vi "JKI_Python_Server Example 2 Nodes.vi"() -> ()   [LabVIEW 2013]
uses:
  Server/Type Definitions/Python Method.ctl
  Server/Register for Events (Single PyObject).vi
  Server/Server.lvclass
  Call/Call.lvclass
panel:
  out "Number of Connections":u32
  out "Client Connected":bool
  out "error out":errorcluster
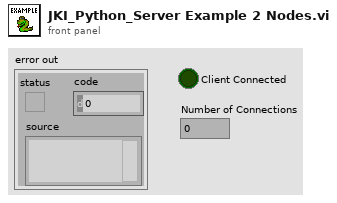
[diagram p1: front panel]
types:
  T1 = typedef "JKI_Python_Bridge_for_LV.lvlib/Server.lvclass/Python Method.ctl" = cluster{"Name":string, "Arguments":string[], "Documentation":string}
  T2 = typedef "JKI_Python_Bridge_for_LV.lvlib/Server.lvclass/Python Method Call - Event Registration.ctl" = refnum<event-registration>
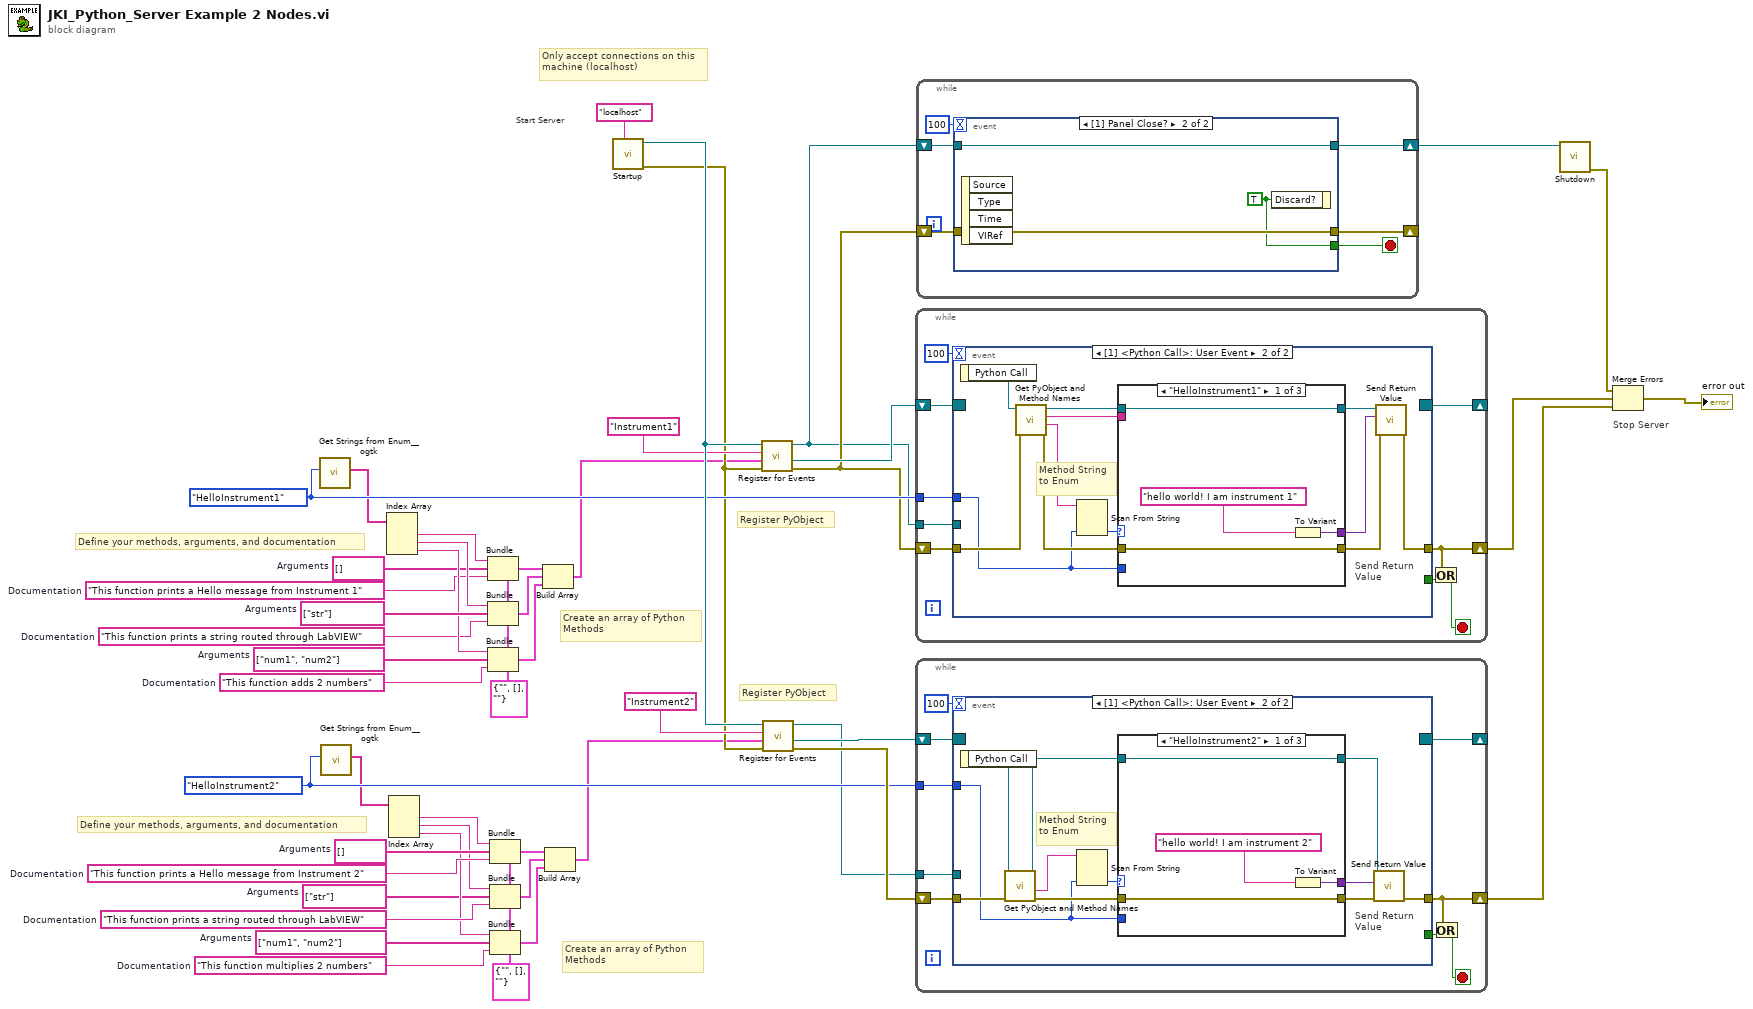
[diagram p0: block diagram]
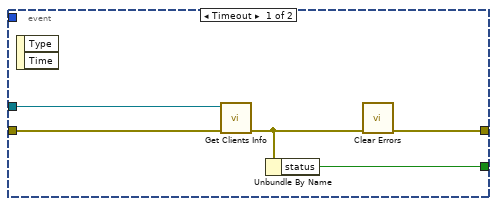
[diagram p2: hidden frame]
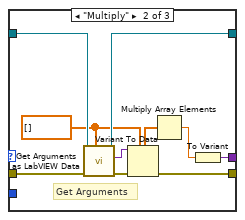
[diagram p3: hidden frame]
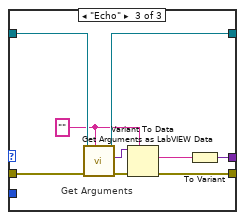
[diagram p4: hidden frame]
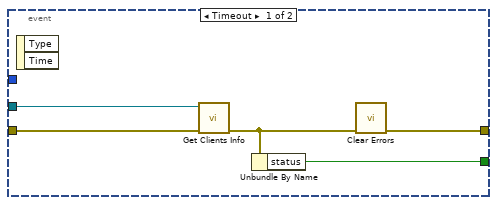
[diagram p5: hidden frame]
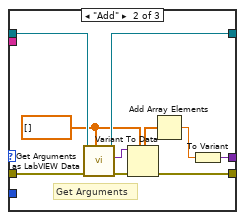
[diagram p6: hidden frame]
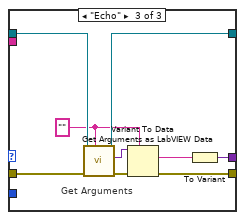
[diagram p7: hidden frame]
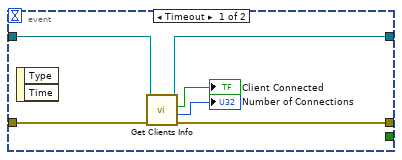
[diagram p8: hidden frame]
diagram:
  w15 = string[] []  # Arguments
  w14 = T1 {"Name"="", "Arguments"=[], "Documentation"=""} ("Method")
  w13 = "This function multiplies 2 numbers"  # Documentation
  w12 = "This function prints a string routed through LabVIEW"  # Documentation
  w11 = "This function prints a Hello message from Instrument 2"  # Documentation
  w6 = string[] ["num1", "num2"]  # Arguments
  w5 = string[] ["str"]  # Arguments
  w18 = string[] []  # Arguments
  w19 = T1 {"Name"="", "Arguments"=[], "Documentation"=""} ("Method")
  w20 = "This function adds 2 numbers"  # Documentation
  w21 = "This function prints a string routed through LabVIEW"  # Documentation
  w22 = "This function prints a Hello message from Instrument 1"  # Documentation
  w27 = string[] ["num1", "num2"]  # Arguments
  w28 = string[] ["str"]  # Arguments
  w40 = enum16{"HelloInstrument2", "Echo", "Multiply"}."HelloInstrument2"
  w39 = enum16{"HelloInstrument1", "Echo", "Add"}."HelloInstrument1"
  # "Create an array of Python \nMethods"
  # "Define your methods, arguments, and documentation"
  # "Create an array of Python \nMethods"
  # "Define your methods, arguments, and documentation"
  # "Register PyObject"
  # "Register PyObject"
  # "Stop Server"
  # "Start Server"
  # "Only accept connections on this machine (localhost)"
  n1 = call <userlib>:"Get Strings from Enum__ogtk.vi"("Enum"=w39) -> ("Enum Strings"=w17:string[])  [unwired: 7 in, 3 out]
  n2 = call <userlib>:"Get Strings from Enum__ogtk.vi"("Enum"=w40) -> ("Enum Strings"=w2:string[])  [unwired: 7 in, 3 out]
  n3 = Index Array(array=w17) -> (element #1=w30:string, element #2=w29:string, element #3=w26:string)  [unwired: 3 in]
  n4 = Index Array(array=w2) -> (element #1=w3:string, element #2=w4:string, element #3=w7:string)  [unwired: 3 in]
  n5 = Bundle(cluster=w19, "Name"=w30, "Arguments"=w18, "Documentation"=w22) -> (w25:T1)
  n6 = Bundle(cluster=w19, "Name"=w29, "Arguments"=w28, "Documentation"=w21) -> (w24:T1)
  n7 = Bundle(cluster=w19, "Name"=w26, "Arguments"=w27, "Documentation"=w20) -> (w23:T1)
  n8 = Bundle(cluster=w14, "Name"=w3, "Arguments"=w15, "Documentation"=w11) -> (w8:T1)
  n9 = Bundle(cluster=w14, "Name"=w4, "Arguments"=w5, "Documentation"=w12) -> (w9:T1)
  n10 = Bundle(cluster=w14, "Name"=w7, "Arguments"=w6, "Documentation"=w13) -> (w10:T1)
  n11 = Build Array(w25, w24, w23) -> (w16:T1[])
  n12 = Build Array(w8, w9, w10) -> (w1:T1[])
  n13 = call "Startup.vi"("IP Address (localhost)"="localhost" ("name")) -> ("error out"=w35:errorcluster, "JKI_Python_Server out"=w47:refnum<class "Server.lvclass">)  [unwired: 9 in]
  n14 = call-poly "Register for Events.vi"("error in (no error)"=w35, "Functions"=w16, "PyObject Name"="Instrument1" ("Python Node Name"), "JKI_Python_Server in"=w47) -> ("error out"=w38:errorcluster, "Python"=w41:T2, "JKI_Python_Server out"=w34:refnum<class "Server.lvclass">)  [unwired: 5 in]
  n15 = call-poly "Register for Events.vi"("error in (no error)"=w35, "Functions"=w1, "PyObject Name"="Instrument2" ("Python Node Name"), "JKI_Python_Server in"=w47) -> ("error out"=w43:errorcluster, "Python"=w42:T2, "JKI_Python_Server out"=w33:refnum<class "Server.lvclass">)  [unwired: 5 in]
  n16 = while {
    shift-right: [w51] -> w44
    shift-left: w38 -> [w56]
    shift-right: [w54] -> _
    shift-left: w41 -> [w57]
    tunnel: w39 -> [w53]
    tunnel: w34 -> [w52]
    stop <- w50 stop-if-true
    n17 = event shown="[1] <Python Call>: User Event" {
      selector: w57 -> [_ _]
      dyn-events: [_ _] -> w54
      timeout: 100 -> [_ _]
      tunnel: [w58 w67] -> w51
      tunnel: w56 -> [w62 w72]
      tunnel: w53 -> [_ w69]
      tunnel: w52 -> [w61 _]
      tunnel: [w59 _] -> w49
      event Timeout {
        n18 = event-data() -> ()  [unwired: 1 in, 2 out]
        n19 = call "Get Clients Info.vi"("error in (no error)"=w62, "JKI_Python_Server in"=w61) -> ("error out"=w60:errorcluster)  [unwired: 5 in, 4 out]
        n20 = Unbundle By Name(w60) -> ("status"=w59:bool)
        n21 = call <vilib>:"Clear Errors.vi"("error in (no error)"=w60) -> ("error out"=w58:errorcluster)  [unwired: 6 in]
      }
      event User Event {
        # "Send Return\nValue"
        # "Method String to Enum"
        n22 = event-data() -> ("Python Call"=w73:refnum<class "Call.lvclass">)  [unwired: 1 in]
        n23 = call "Get PyObject and Method Names.vi"("error in (no error)"=w72, "Call in"=w73) -> ("error out"=w71:errorcluster, "Method Name"=w64:string, "PyObject Name"=w63:string, "Call out"=w70:refnum<class "Call.lvclass">)  [unwired: 6 in]
        n24 = Scan From String(input string=w64, default 1=w69) -> (output 1=w74:enum16{"HelloInstrument1", "Echo", "Add"})  [unwired: 3 in, 3 out]
        n25 = case shown="\"HelloInstrument1\"" w74 {
          tunnel: [w75 w79 w89] -> w66
          tunnel: w71 -> [w77 w82 w93]
          tunnel: [w77 w87 w97] -> w68
          tunnel: [w76 w84 w95] -> w65
          tunnel: w70 -> [w76 w85 w96]
          tunnel: w69 -> [_ _ _]
          tunnel: w63 -> [_ _ _]
          frame "HelloInstrument1" {
            n26 = To Variant(anything="hello world! I am instrument 1" ("Arguments")) -> (Variant=w75:variant)
          }
          frame "Add" {
            w80 = dbl[] []
            # "Get Arguments"
            n27 = call "Get Arguments as LabVIEW Data.vi"("type"=w80, "error in (no error)"=w82, "Call in"=w85) -> ("error out"=w81:errorcluster, "LabVIEW Data"=w83:variant, "Call out"=w84:refnum<class "Call.lvclass">)  [unwired: 6 in]
            n28 = Variant To Data(error in=w81, type=w80, Variant=w83) -> (data=w88:dbl[], error out=w87:errorcluster)
            n29 = Add Array Elements(numeric array=w88) -> (sum=w86:dbl)
            n30 = To Variant(anything=w86) -> (Variant=w79:variant)
          }
          frame "Echo" {
            w91 = ""
            # "Get Arguments"
            n31 = call "Get Arguments as LabVIEW Data.vi"("type"=w91, "error in (no error)"=w93, "Call in"=w96) -> ("error out"=w92:errorcluster, "LabVIEW Data"=w94:variant, "Call out"=w95:refnum<class "Call.lvclass">)  [unwired: 6 in]
            n32 = Variant To Data(error in=w92, type=w91, Variant=w94) -> (data=w90:string, error out=w97:errorcluster)
            n33 = To Variant(anything=w90) -> (Variant=w89:variant)
          }
        }
        n34 = call "Send Return Value.vi"("error in (no error)"=w68, "Return Value"=w66, "Response in"=w65) -> ("error out"=w67:errorcluster)  [unwired: 8 in]
      }
    }
    n35 = Or(x=w51, y=w49) -> (x .or. y?=w50:bool)
  }
  n36 = while {
    shift-right: [w100] -> w45
    shift-left: w43 -> [w105]
    shift-right: [w103] -> _
    shift-left: w42 -> [w106]
    tunnel: w40 -> [w102]
    tunnel: w33 -> [w101]
    stop <- w99 stop-if-true
    n37 = event shown="[1] <Python Call>: User Event" {
      selector: w106 -> [_ _]
      dyn-events: [_ _] -> w103
      timeout: 100 -> [_ _]
      tunnel: [w107 w114] -> w100
      tunnel: w105 -> [w111 w120]
      tunnel: w102 -> [_ w117]
      tunnel: w101 -> [w110 _]
      tunnel: [w108 _] -> w98
      event Timeout {
        n38 = event-data() -> ()  [unwired: 1 in, 2 out]
        n39 = call "Get Clients Info.vi"("error in (no error)"=w111, "JKI_Python_Server in"=w110) -> ("error out"=w109:errorcluster)  [unwired: 5 in, 4 out]
        n40 = Unbundle By Name(w109) -> ("status"=w108:bool)
        n41 = call <vilib>:"Clear Errors.vi"("error in (no error)"=w109) -> ("error out"=w107:errorcluster)  [unwired: 6 in]
      }
      event User Event {
        # "Send Return\nValue"
        # "Method String to Enum"
        n42 = event-data() -> ("Python Call"=w121:refnum<class "Call.lvclass">)  [unwired: 1 in]
        n43 = call "Get PyObject and Method Names.vi"("error in (no error)"=w120, "Call in"=w121) -> ("error out"=w119:errorcluster, "Method Name"=w116:string, "Call out"=w118:refnum<class "Call.lvclass">)  [unwired: 6 in, 1 out]
        n44 = Scan From String(input string=w116, default 1=w117) -> (output 1=w122:enum16{"HelloInstrument2", "Echo", "Multiply"})  [unwired: 3 in, 3 out]
        n45 = case shown="\"HelloInstrument2\"" w122 {
          tunnel: [w123 w127 w137] -> w113
          tunnel: w119 -> [w125 w130 w141]
          tunnel: [w125 w135 w145] -> w115
          tunnel: [w124 w132 w143] -> w112
          tunnel: w118 -> [w124 w133 w144]
          tunnel: w117 -> [_ _ _]
          frame "HelloInstrument2" {
            n46 = To Variant(anything="hello world! I am instrument 2" ("Arguments")) -> (Variant=w123:variant)
          }
          frame "Multiply" {
            w128 = dbl[] []
            # "Get Arguments"
            n47 = call "Get Arguments as LabVIEW Data.vi"("type"=w128, "error in (no error)"=w130, "Call in"=w133) -> ("error out"=w129:errorcluster, "LabVIEW Data"=w131:variant, "Call out"=w132:refnum<class "Call.lvclass">)  [unwired: 6 in]
            n48 = Variant To Data(error in=w129, type=w128, Variant=w131) -> (data=w136:dbl[], error out=w135:errorcluster)
            n49 = Multiply Array Elements(1:w136) -> (0:w134:dbl)
            n50 = To Variant(anything=w134) -> (Variant=w127:variant)
          }
          frame "Echo" {
            w139 = ""
            # "Get Arguments"
            n51 = call "Get Arguments as LabVIEW Data.vi"("type"=w139, "error in (no error)"=w141, "Call in"=w144) -> ("error out"=w140:errorcluster, "LabVIEW Data"=w142:variant, "Call out"=w143:refnum<class "Call.lvclass">)  [unwired: 6 in]
            n52 = Variant To Data(error in=w140, type=w139, Variant=w142) -> (data=w138:string, error out=w145:errorcluster)
            n53 = To Variant(anything=w138) -> (Variant=w137:variant)
          }
        }
        n54 = call "Send Return Value.vi"("error in (no error)"=w115, "Return Value"=w113, "Response in"=w112) -> ("error out"=w114:errorcluster)  [unwired: 8 in]
      }
    }
    n55 = Or(x=w100, y=w98) -> (x .or. y?=w99:bool)
  }
  n56 = while {
    shift-right: [w147] -> _
    shift-left: w38 -> [w151]
    shift-right: [w148] -> w46
    shift-left: w34 -> [w149]
    stop <- w146 stop-if-true
    n57 = event shown="[1] Panel Close?" {
      selector: _ -> [_ _]
      dyn-events: _ -> [_ _]
      timeout: 100 -> [_ _]
      tunnel: [w155 w160] -> w147
      tunnel: w151 -> [w156 w160]
      tunnel: w149 -> [w157 w159]
      tunnel: [w154 w159] -> w148
      tunnel: [_ w158] -> w146
      event Timeout {
        n58 = event-data() -> ()  [unwired: 1 in, 2 out]
        n59 = call "Get Clients Info.vi"("error in (no error)"=w156, "JKI_Python_Server in"=w157) -> ("error out"=w155:errorcluster, "Number of Connections"=→"Number of Connections":u32, "Client Connected"=→"Client Connected":bool, "JKI_Python_Server out"=w154:refnum<class "Server.lvclass">)  [unwired: 5 in, 1 out]
      }
      event Panel Close? {
        w158 = TRUE ("Discard?")
        n60 = event-data() -> ()  [unwired: 1 in, 4 out]
        n61 = event-data("Discard?"=w158) -> ()  [unwired: 1 in, 1 out]
      }
    }
  }
  n62 = call "Shutdown.vi"("JKI_Python_Server in"=w46) -> ("error out"=w32:errorcluster)  [unwired: 10 in]
  n63 = Merge Errors(w32, w44, w45) -> (→"error out":errorcluster)
